vi "Command Drive Time.vi"(7 "Startup":bool, 9 "Translation (Throttle)":dbl, 10 "Drive (Throttle)":dbl, 11 "Time to Run (ms)":dbl) -> (2 "Right Wheel":dbl, 3 "Left Wheel":dbl, 4 "Reinit":bool, 6 "Completed":bool)   [LabVIEW 2019]
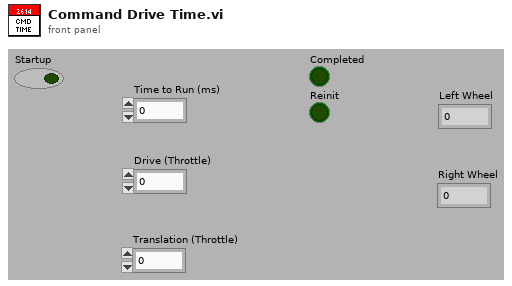
[diagram p1: front panel]
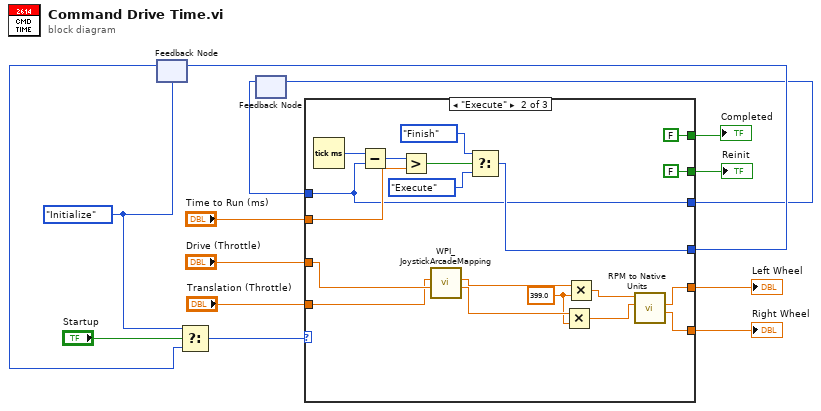
[diagram p0: block diagram]
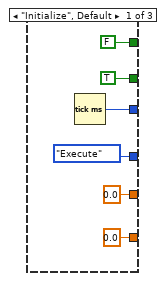
[diagram p2: hidden frame]
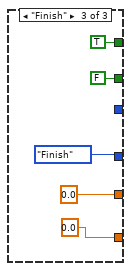
[diagram p3: hidden frame]
diagram:
  w12 = enum16{"Initialize", "Execute", "Finish"}."Initialize"
  n1 = feedback #1(w12) -> (w7:enum16{"Initialize", "Execute", "Finish"})
  n2 = Select(t=w12, s="Startup", f=w7) -> (s? t:f=w13:enum16{"Initialize", "Execute", "Finish"})
  n3 = feedback #2() -> (w6:u32)  [unwired: 1 in]
  n4 = case shown="\"Execute\"" w13 {
    tunnel: [FALSE FALSE TRUE] -> w11
    tunnel: [TRUE FALSE FALSE] -> w10
    tunnel: [enum16{"Initialize", "Execute", "Finish"}."Execute" w31 enum16{"Initialize", "Execute", "Finish"}."Finish"] -> w9
    tunnel: [w17 w30 _] -> w8
    tunnel: w6 -> [_ w30 _]
    tunnel: "Time to Run (ms)" -> [_ w34 _]
    tunnel: [0.0 ("Left Wheel Velocity") w22 0.0] -> w4
    tunnel: [0.0 ("Right Wheel Velocity") w21 0.0] -> w3
    tunnel: "Drive (Throttle)" -> [_ w29 _]
    tunnel: "Translation (Throttle)" -> [_ w28 _]
    frame "Initialize", Default {
      n5 = Tick Count (ms)() -> (millisecond timer value=w17:u32)
    }
    frame "Execute" {
      w25 = 399.0 ("y")
      n6 = Tick Count (ms)() -> (millisecond timer value=w37:u32)
      n7 = Subtract(x=w37, y=w30) -> (x-y=w38:u32)
      n8 = Greater?(x=w38, y=w34) -> (0:w39:bool)
      n9 = call <vilib>:"WPI_JoystickArcadeMapping.vi"("Y axis value"=w29, "X axis value"=w28) -> ("Right Motor Value"=w26:dbl, "Left Motor Value"=w27:dbl)  [unwired: 8 in]
      n10 = Select(t=enum16{"Initialize", "Execute", "Finish"}."Finish", s=w39, f=enum16{"Initialize", "Execute", "Finish"}."Execute") -> (s? t:f=w31:enum16{"Initialize", "Execute", "Finish"})
      n11 = Multiply(x=w26, y=w25) -> (x*y=w23:dbl)
      n12 = Multiply(x=w27, y=w25) -> (x*y=w24:dbl)
      n13 = call "RPM to Native Units.vi"("Right RPM"=w23, "Left RPM"=w24) -> ("Right Out"=w21:dbl, "Left Out"=w22:dbl)  [unwired: 6 in, 1 out]
    }
    frame "Finish" {
    }
  }
  "Completed" <- w11
  "Reinit" <- w10
  "Left Wheel" <- w4
  "Right Wheel" <- w3
  n14 = feedback-in #1(w9) -> ()
  n15 = feedback-in #2(w8) -> ()
